vi "globals.vi"() -> ()   [LabVIEW 2020, in "Netatmo-WeatherStation.lvlib"]
uses:
  Netatmo-WeatherStation.lvlib
panel:
  in  "password":string
  in  "username":string
  in  "expire_time":timestamp
  in  "refresh_token":string
  in  "access_token":string
  in  "grant_type":string
  in  "getstationsdata uri":string="https://api.netatmo.com/api/getstationsdata"
  in  "device_id":string="70:ee:50:02:b8:74"
  in  "token request uri":string="https://api.netatmo.com/oauth2/token "
  in  "client secret":string="nZJjw6391sswie2Kj0fKIysFXknN"
  in  "scope":string="read_station"
  in  "authorization endpoint":string="https://api.netatmo.com/oauth2/authorize"
  in  "client id":string="5fc26e350dda4328cf4129e5"
  in  "redirect uri":string="http://127.0.0.1:8001/OAuth/Redirect"
  out "Events":T1
  in  "Redirection HTML":string="<html>\n<head><meta http-equiv='refresh' content='5;url=https://my.netatmo.com/app/station'></head>\n<body>Please return to the app.</body>\n</html>"
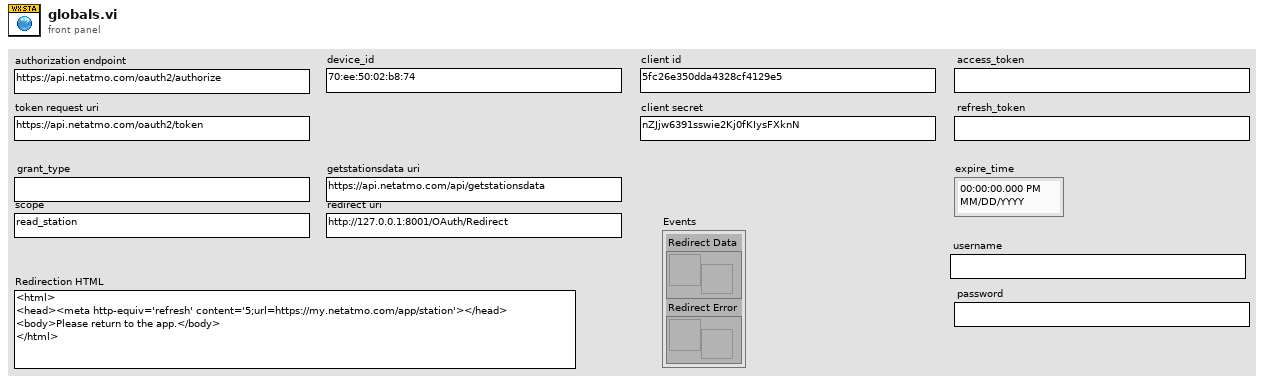
[diagram p1: front panel]
types:
  T1 = cluster{"Redirect Data":refnum<user-event>, "Redirect Error":refnum<user-event>}
diagram:
